vi "LabVIEW_ArduinoControls_TimeProtoType.vi"() -> ()   [LabVIEW 2021]
uses:
  <vilib>/Instr/_visa.llb/VISA Configure Serial Port (Instr).vi
panel:
  out "Horz Distance":dbl(graph)
  out "RPM":dbl(graph)
  out "Vertical Motor Speed":dbl(graph)
  out "Vertical Distance":dbl(graph)
  out "Weight on Bit":dbl(graph)
  out "System Amps":dbl(graph)
  out "RPM":cluster{"X":dbl, "Y":dbl}[](graph)
  out "System Amps":cluster{"X":dbl, "Y":dbl}[](graph)
  out "Horz Distance":cluster{"X":dbl, "Y":dbl}[](graph)
  out "Vertical Distance":cluster{"X":dbl, "Y":dbl}[](graph)
  out "Vertical Motor Speed":cluster{"X":dbl, "Y":dbl}[](graph)
  out "Weight on Bit":cluster{"X":dbl, "Y":dbl}[](graph)
  in  "DRILL STOP":bool
  in  "Drill Speed Arduino 2.0 Write Stop":bool
  in  "Slow Down":bool
  in  "Speed Up":bool
  in  "Drill Speed Arduino 2 Write":refnum<visa-resource-name>
  in  "Stepper Arduino 1 Serial Read":refnum<visa-resource-name>
  out "Data Packet Arduini 1 Matched":i32
  in  "Arduino 1.0 Read Stop":bool
  in  "Arduino 2.0 Read Stop":bool
  in  "Emergency Stop! 3":bool
  in  "Emergency Stop! 2":bool
  in  "GO DOWN 3":bool
  in  "GO DOWN 2":bool
  in  "GO UP 3":bool
  in  "GO UP 2":bool
  in  "MAX SPEED 3":bool
  in  "MAX SPEED 2":bool
  in  "SLOWEST SPEED 3":bool
  in  "SLOWEST SPEED 2":bool
  in  "Decellerate 3":bool
  in  "Decellerate 2":bool
  in  "Accelerate 3":bool
  in  "Accelerate 2":bool
  in  "Drill Speed Arduino 2 Serial Read":refnum<visa-resource-name>
  out "Data Packet Received":i32
  in  "GO UP":bool
  in  "GO DOWN":bool
  in  "MAX SPEED":bool
  in  "SLOWEST SPEED":bool
  out "concatenated string":string
  in  "Arduino 1.0 Write Stop":bool
  in  "Emergency Stop!":bool
  in  "Decellerate":bool
  in  "Stepper Arduino 1 Write":refnum<visa-resource-name>
  in  "Accelerate":bool
  # "Drill Speed Controls"
  # "WINCH CONTROLS"
  # "VERTICAL STEPPER MOTOR CONTROLS"
  # "HORIZONTAL STEPPER MOTOR CONTROLS"
  # "-1 Means Not Found\nany value greater than 0 corresponds to the amount\nof matching characters found"
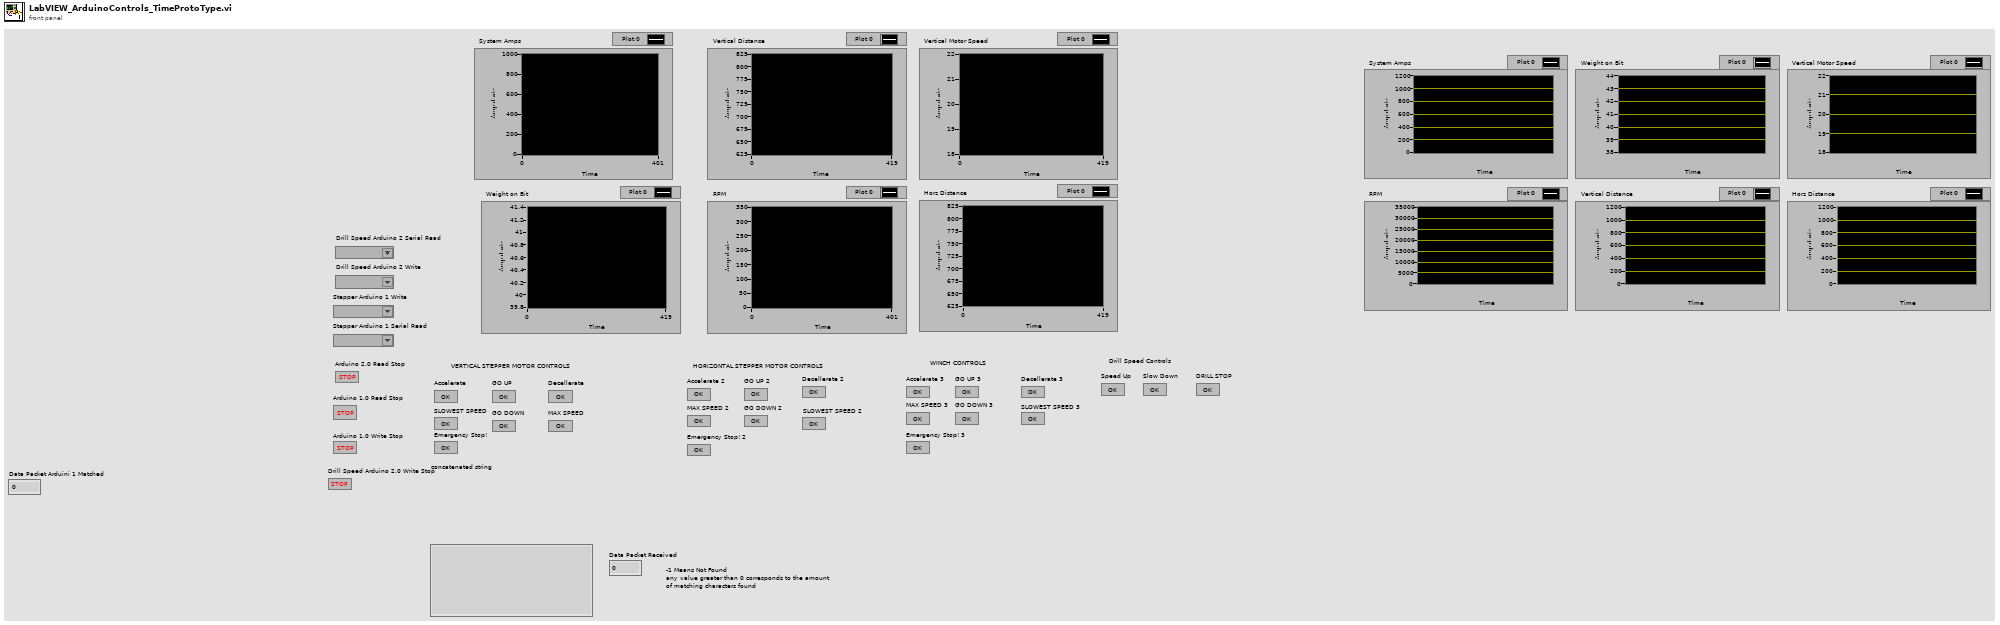
[diagram p1: front panel]
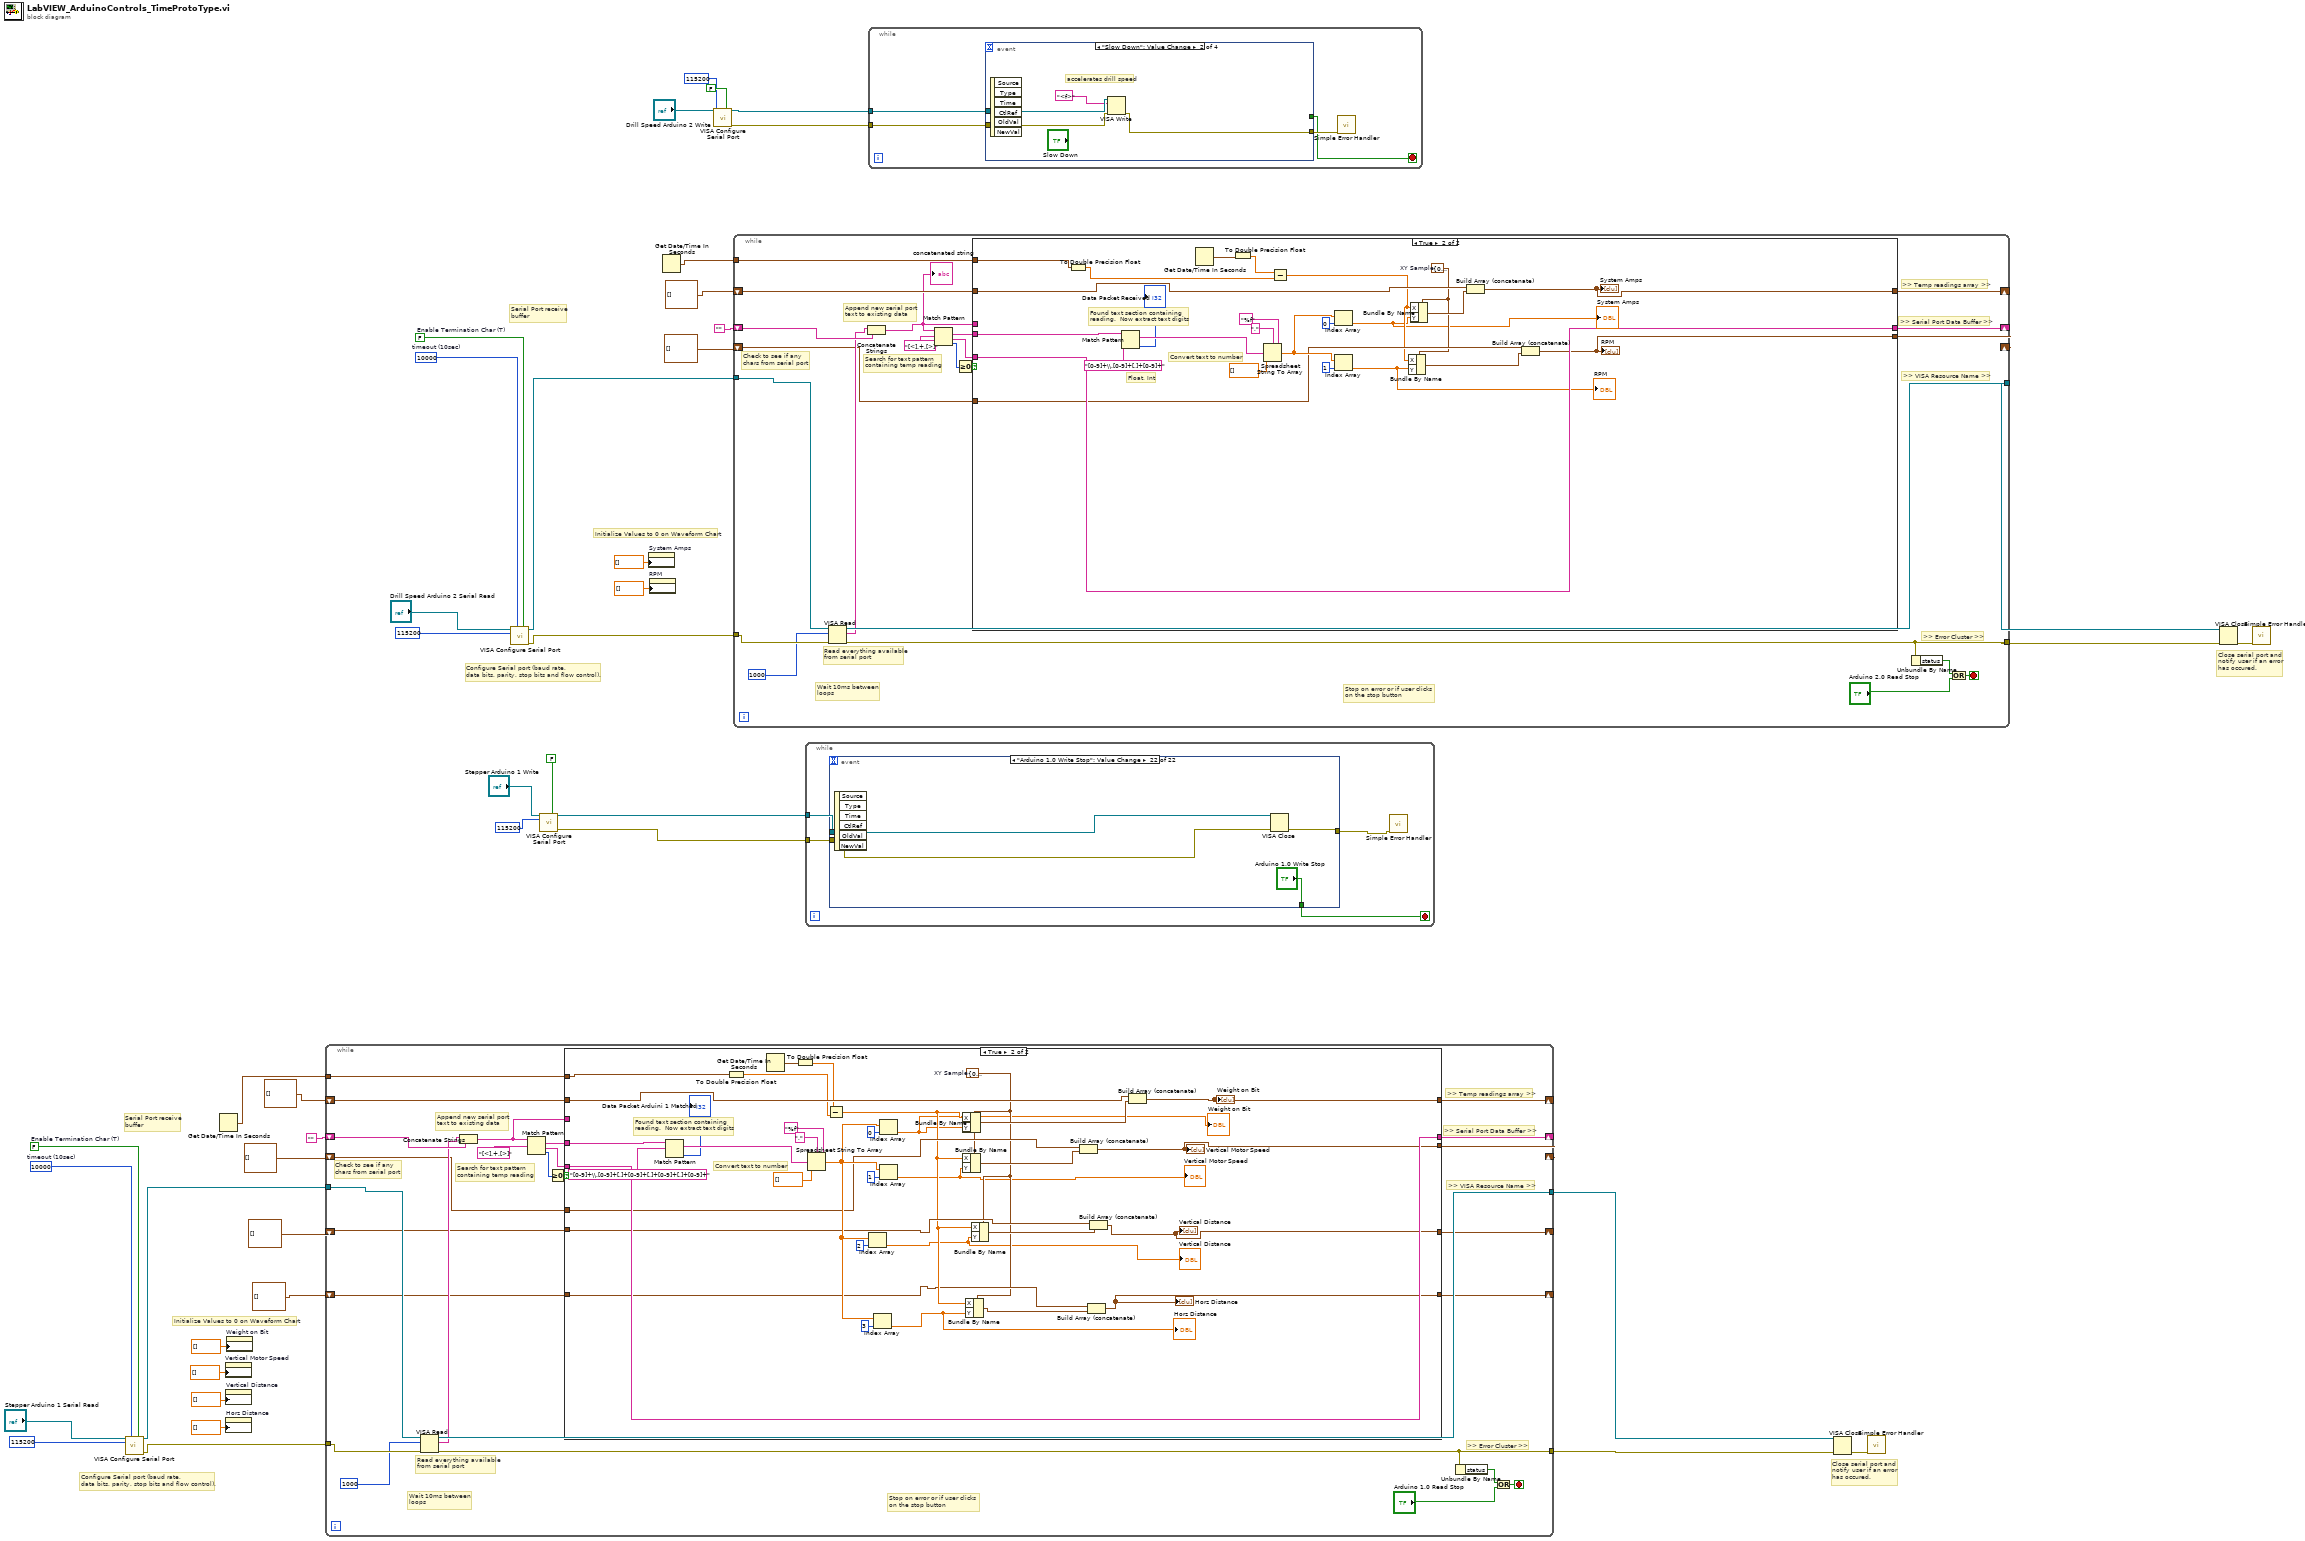
[diagram p0: block diagram]
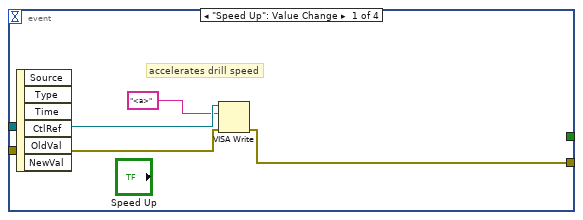
[diagram p2: hidden frame]
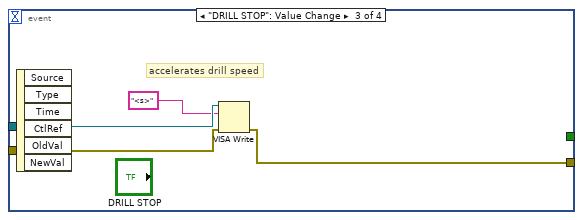
[diagram p3: hidden frame]
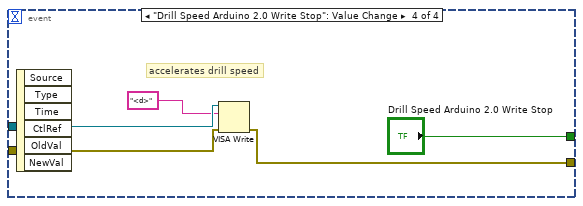
[diagram p4: hidden frame]
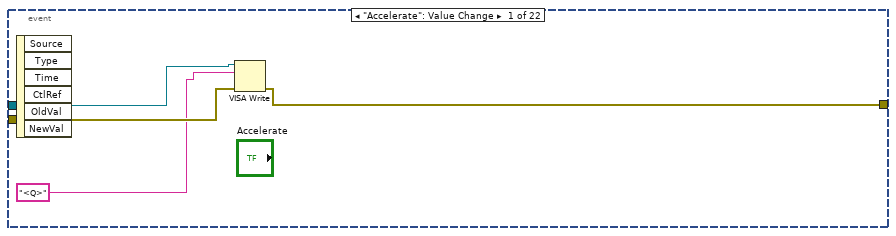
[diagram p7: hidden frame]
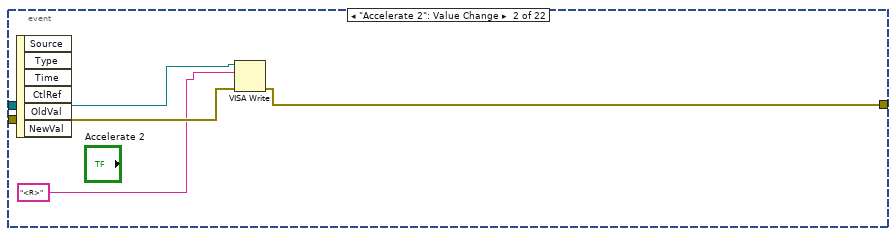
[diagram p8: hidden frame]
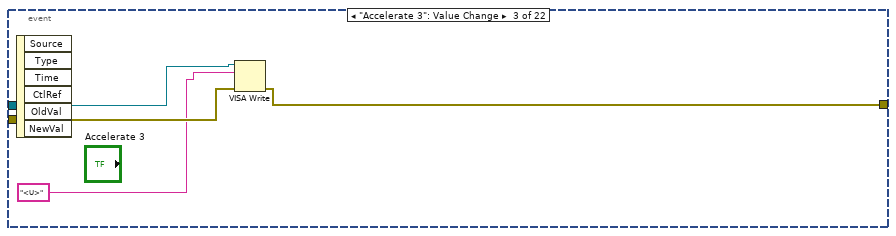
[diagram p9: hidden frame]
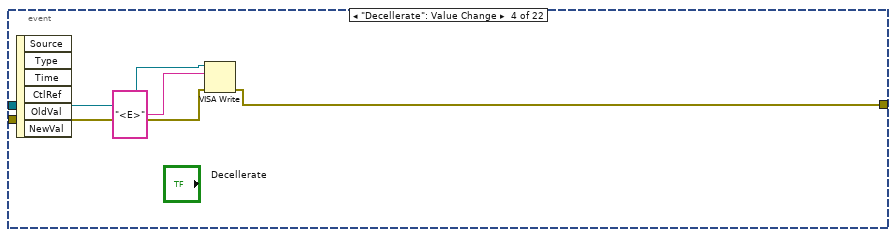
[diagram p10: hidden frame]
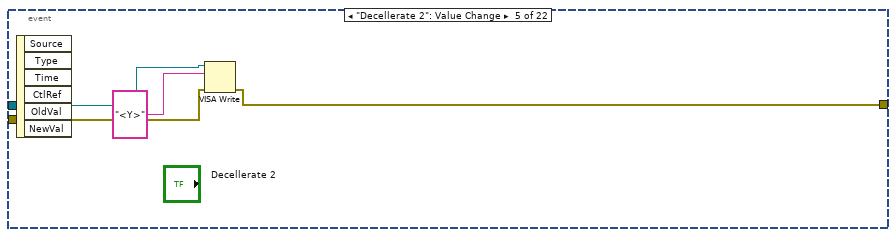
[diagram p11: hidden frame]
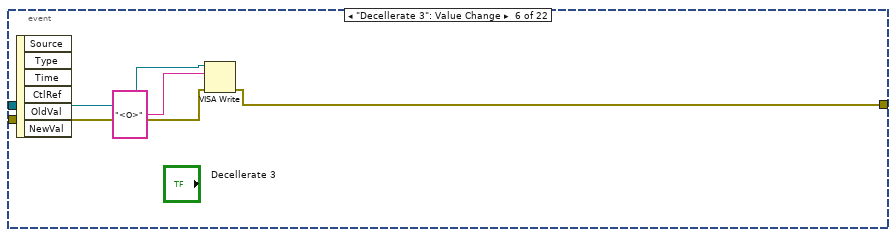
[diagram p12: hidden frame]
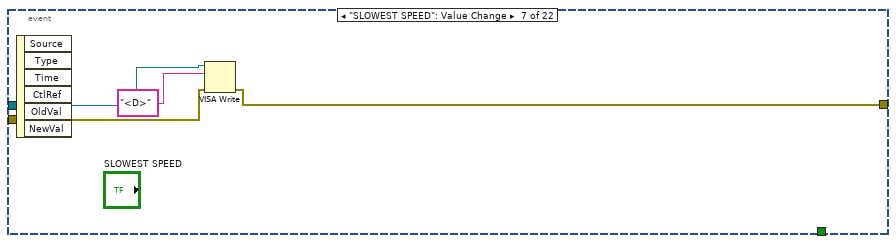
[diagram p13: hidden frame]
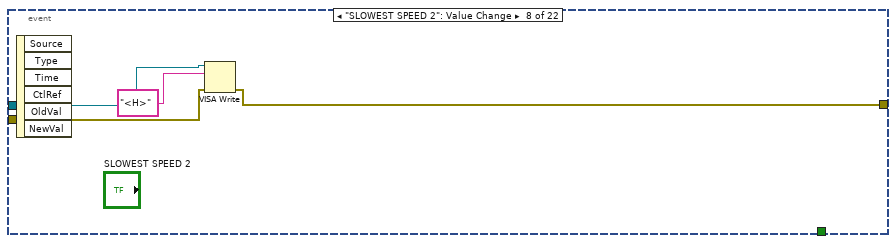
[diagram p14: hidden frame]
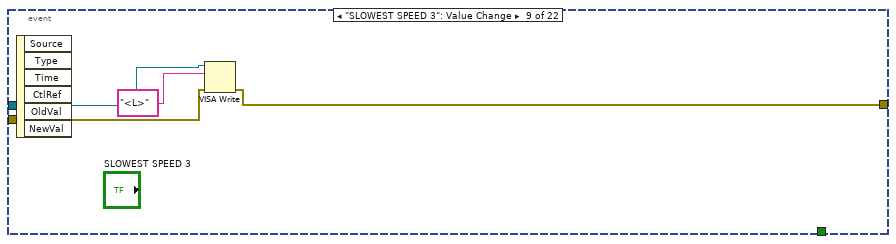
[diagram p15: hidden frame]
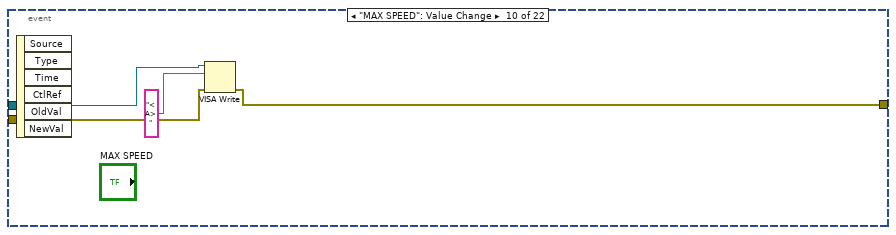
[diagram p16: hidden frame]
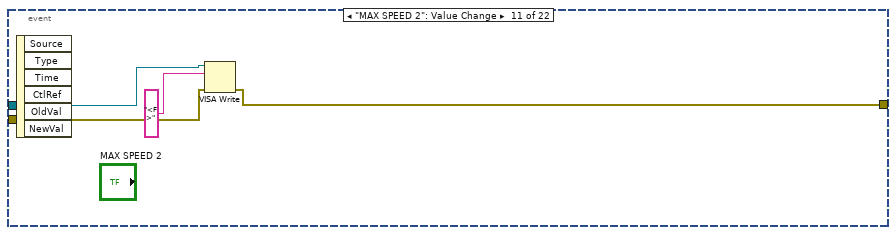
[diagram p17: hidden frame]
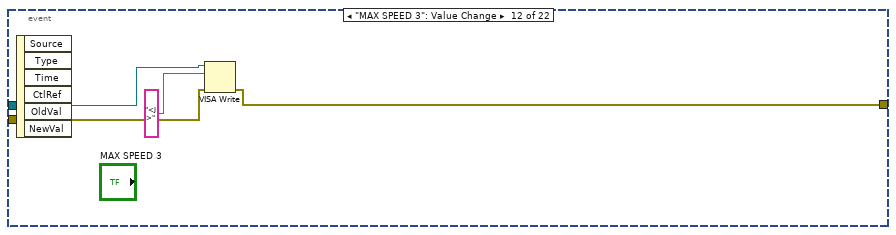
[diagram p18: hidden frame]
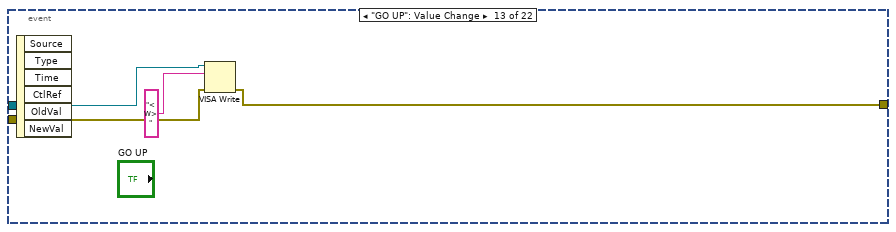
[diagram p19: hidden frame]
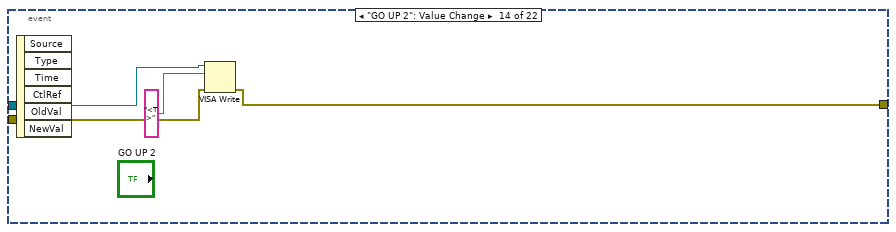
[diagram p20: hidden frame]
diagram:
  w25 = FALSE  # Enable Termination Char (T)
  w26 = u32 10000  # timeout (10sec)
  w36 = FALSE  # Enable Termination Char (T)
  w37 = u32 10000  # timeout (10sec)
  # "Initialize Values to 0 on Waveform Chart"
  # "Initialize Values to 0 on Waveform Chart"
  # "Close serial port and\nnotify user if an error\nhas occured."
  # "Serial Port receive\nbuffer"
  # "Configure Serial port (baud rate,\ndata bits, parity, stop bits and flow control)."
  # "Close serial port and\nnotify user if an error\nhas occured."
  # "Serial Port receive\nbuffer"
  # "Configure Serial port (baud rate,\ndata bits, parity, stop bits and flow control)."
  n1 = call-poly "VISA Configure Serial Port"("VISA resource name"="Stepper Arduino 1 Serial Read", "timeout (10sec)"=w26, "Enable Termination\nChar (T)"=w25, "baud rate (9600)"=u32 115200) -> ("VISA resource name out"=w22:refnum<visa-resource-name>, "error out"=w21:errorcluster)  [unwired: 10 in]
  n2 = Get Date/Time In Seconds() -> (seconds since 1Jan1904=w13:timestamp)
  n3 = property on="Vertical Motor Speed" class="WFChart (strict)"("History Data"=dbl[] []) -> ()  [unwired: 2 in, 2 out]
  n4 = property on="Vertical Distance" class="WFChart (strict)"("History Data"=dbl[] []) -> ()  [unwired: 2 in, 2 out]
  n5 = property on="Horz Distance" class="WFChart (strict)"("History Data"=dbl[] []) -> ()  [unwired: 2 in, 2 out]
  n6 = property on="Weight on Bit" class="WFChart (strict)"("History Data"=dbl[] []) -> ()  [unwired: 2 in, 2 out]
  n7 = while {
    tunnel: [w68] -> w29
    tunnel: [w70] -> w28
    shift-right: [w63] -> _
    shift-left: "" -> [w69]
    shift-right: [w65] -> _
    shift-left: cluster{"X":dbl, "Y":dbl}[] [] ("XY Graph") -> [w64]
    tunnel: w22 -> [w62]
    tunnel: w21 -> [w61]
    shift-right: [w53] -> _
    shift-left: cluster{"X":dbl, "Y":dbl}[] [] ("XY Graph") -> [w52]
    shift-right: [w48] -> _
    shift-left: cluster{"X":dbl, "Y":dbl}[] [] ("XY Graph") -> [w49]
    shift-right: [w46] -> _
    shift-left: cluster{"X":dbl, "Y":dbl}[] [] ("XY Graph") -> [w47]
    tunnel: w13 -> [w45]
    stop <- w67 stop-if-true
    # "Search for text pattern\ncontaining temp reading"
    # "Append new serial port\ntext to existing data"
    # "Read everything available\nfrom serial port"
    # "Wait 10ms between \nloops"
    # "Stop on error or if user clicks \non the stop button"
    # ">> Error Cluster >>"
    # ">> VISA Resource Name >>"
    # ">> Temp readings array >>"
    # ">> Serial Port Data Buffer >>"
    # "Check to see if any\nchars from serial port"
    n8 = VISA Read(VISA resource name=w62, byte count=u32 1000, error in (no error)=w61) -> (VISA resource name out=w70:refnum<visa-resource-name>, read buffer=w55:string, error out=w68:errorcluster)  [unwired: 1 out]
    n9 = Concatenate Strings(w55, w69) -> (w50:string)
    n10 = Match Pattern(string=w50, regular expression="[<].+.[>]") -> (match substring=w57:string, after substring=w56:string, offset past match=w59:i32)  [unwired: 1 in, 1 out]
    n11 = Greater Or Equal To 0?(x=w59) -> (x >= 0?=w58:bool)
    n12 = case shown="True" w58 {
      tunnel: w57 -> [_ w109]
      tunnel: w56 -> [_ w110]
      tunnel: [w73 w110] -> w63
      tunnel: [w75 w96] -> w65
      tunnel: w64 -> [w75 w97]
      tunnel: [w74 w90] -> w53
      tunnel: w52 -> [w74 w89]
      tunnel: w50 -> [w73 _]
      tunnel: w49 -> [w72 w86]
      tunnel: [w72 w87] -> w48
      tunnel: w47 -> [w71 w83]
      tunnel: [w71 w80] -> w46
      tunnel: w45 -> [_ w95]
      frame False {
        # "Did not find text pattern in the buffer.  Try again in the next loop after new data \nhas been received."
      }
      frame True {
        w81 = cluster{"X":dbl, "Y":dbl} {"X"=0.0, "Y"=0.0}  # XY Sample
        # "Convert text to number"
        # "Found text section containing \nreading.  Now extract text digits"
        n13 = Match Pattern(string=w109, regular expression="[0-9]+\\.[0-9]+[,]+[0-9]+[,]+[0-9]+[,]+[0-9]+") -> (match substring=w103:string, offset past match=→"Data Packet Arduini 1 Matched":i32)  [unwired: 1 in, 2 out]
        n14 = To Double Precision Float(number=w95) -> (double precision float=w94:dbl)
        n15 = Get Date/Time In Seconds() -> (seconds since 1Jan1904=w93:timestamp)
        n16 = To Double Precision Float(number=w93) -> (double precision float=w92:dbl)
        n17 = Spreadsheet String To Array(delimiter (Tab)=",", format string="%f", spreadsheet string=w103, array type (2D Dbl)=dbl[] []) -> (array=w99:dbl[])
        n18 = Subtract(x=w92, y=w94) -> (x-y=w84:dbl)
        n19 = Index Array(array=w99, index=2) -> (element=w77:dbl)
        "Vertical Distance" <- w77
        n20 = Index Array(array=w99, index=3) -> (element=w76:dbl)
        "Horz Distance" <- w76
        n21 = Index Array(array=w99, index=0 ("index (row)")) -> (element=w79:dbl)
        "Weight on Bit" <- w79
        n22 = Index Array(array=w99, index=1 ("index (row)")) -> (element=w78:dbl)
        "Vertical Motor Speed" <- w78
        n23 = Bundle By Name(cluster=w81, "X"=w84, "Y"=w79) -> (w91:cluster{"X":dbl, "Y":dbl})
        n24 = Bundle By Name(cluster=w81, "X"=w84, "Y"=w78) -> (w88:cluster{"X":dbl, "Y":dbl})
        n25 = Bundle By Name(cluster=w81, "X"=w84, "Y"=w76) -> (w82:cluster{"X":dbl, "Y":dbl})
        n26 = Bundle By Name(cluster=w81, "X"=w84, "Y"=w77) -> (w85:cluster{"X":dbl, "Y":dbl})
        n27 = Build Array (concatenate)(w89, w88) -> (w90:cluster{"X":dbl, "Y":dbl}[])
        "Vertical Motor Speed" <- w90
        n28 = Build Array (concatenate)(w83, w82) -> (w80:cluster{"X":dbl, "Y":dbl}[])
        "Horz Distance" <- w80
        n29 = Build Array (concatenate)(w86, w85) -> (w87:cluster{"X":dbl, "Y":dbl}[])
        "Vertical Distance" <- w87
        n30 = Build Array (concatenate)(w97, w91) -> (w96:cluster{"X":dbl, "Y":dbl}[])
        "Weight on Bit" <- w96
      }
    }
    n31 = Unbundle By Name(w68) -> ("status"=w66:bool)
    n32 = Or(x=w66, y="Arduino 1.0 Read Stop") -> (x .or. y?=w67:bool)
  }
  n33 = call-poly "VISA Configure Serial Port"("VISA resource name"="Drill Speed Arduino 2 Serial Read", "timeout (10sec)"=w37, "Enable Termination\nChar (T)"=w36, "baud rate (9600)"=u32 115200) -> ("VISA resource name out"=w33:refnum<visa-resource-name>, "error out"=w32:errorcluster)  [unwired: 10 in]
  n34 = call-poly "VISA Configure Serial Port"("VISA resource name"="Stepper Arduino 1 Write", "Enable Termination\nChar (T)"=FALSE ("Enable Termination\nChar (T)"), "baud rate (9600)"=u32 115200) -> ("VISA resource name out"=w44:refnum<visa-resource-name>, "error out"=w43:errorcluster)  [unwired: 11 in]
  n35 = property on="System Amps" class="WFChart (strict)"("History Data"=dbl[] []) -> ()  [unwired: 2 in, 2 out]
  n36 = property on="RPM" class="WFChart (strict)"("History Data"=dbl[] []) -> ()  [unwired: 2 in, 2 out]
  n37 = Get Date/Time In Seconds() -> (seconds since 1Jan1904=w9:timestamp)
  n38 = call-poly "VISA Configure Serial Port"("VISA resource name"="Drill Speed Arduino 2 Write", "Enable Termination\nChar (T)"=FALSE ("Enable Termination\nChar (T)"), "baud rate (9600)"=u32 115200) -> ("VISA resource name out"=w19:refnum<visa-resource-name>, "error out"=w18:errorcluster)  [unwired: 11 in]
  n39 = while {
    tunnel: [w130] -> w40
    tunnel: [w132] -> w39
    shift-right: [w125] -> _
    shift-left: "" -> [w131]
    shift-right: [w127] -> _
    shift-left: cluster{"X":dbl, "Y":dbl}[] [] ("XY Graph") -> [w126]
    tunnel: w33 -> [w124]
    tunnel: w32 -> [w123]
    shift-right: [w115] -> _
    shift-left: cluster{"X":dbl, "Y":dbl}[] [] ("XY Graph") -> [w114]
    tunnel: w9 -> [w111]
    stop <- w129 stop-if-true
    # "Search for text pattern\ncontaining temp reading"
    # "Append new serial port\ntext to existing data"
    # "Read everything available\nfrom serial port"
    # "Wait 10ms between \nloops"
    # "Stop on error or if user clicks \non the stop button"
    # ">> Error Cluster >>"
    # ">> VISA Resource Name >>"
    # ">> Temp readings array >>"
    # ">> Serial Port Data Buffer >>"
    # "Check to see if any\nchars from serial port"
    n40 = VISA Read(VISA resource name=w124, byte count=u32 1000, error in (no error)=w123) -> (VISA resource name out=w132:refnum<visa-resource-name>, read buffer=w117:string, error out=w130:errorcluster)  [unwired: 1 out]
    n41 = Concatenate Strings(w117, w131) -> (w112:string)
    "concatenated string" <- w112
    n42 = Match Pattern(string=w112, regular expression="[<].+.[>]") -> (match substring=w119:string, after substring=w118:string, offset past match=w121:i32)  [unwired: 1 in, 1 out]
    n43 = Greater Or Equal To 0?(x=w121) -> (x >= 0?=w120:bool)
    n44 = case shown="True" w120 {
      tunnel: w119 -> [_ w159]
      tunnel: w118 -> [_ w160]
      tunnel: [w133 w160] -> w125
      tunnel: [w135 w149] -> w127
      tunnel: w126 -> [w135 w144]
      tunnel: [w134 w142] -> w115
      tunnel: w114 -> [w134 w141]
      tunnel: w112 -> [w133 _]
      tunnel: w111 -> [_ w148]
      frame False {
        # "Did not find text pattern in the buffer.  Try again in the next loop after new data \nhas been received."
      }
      frame True {
        w138 = cluster{"X":dbl, "Y":dbl} {"X"=0.0, "Y"=0.0}  # XY Sample
        # "Float, Int"
        # "Convert text to number"
        # "Found text section containing \nreading.  Now extract text digits"
        n45 = To Double Precision Float(number=w148) -> (double precision float=w146:dbl)
        n46 = Match Pattern(string=w159, regular expression="[0-9]+\\.[0-9]+[,]+[0-9]+") -> (match substring=w153:string, offset past match=→"Data Packet Received":i32)  [unwired: 1 in, 2 out]
        n47 = Get Date/Time In Seconds() -> (seconds since 1Jan1904=w147:timestamp)
        n48 = To Double Precision Float(number=w147) -> (double precision float=w145:dbl)
        n49 = Spreadsheet String To Array(delimiter (Tab)=",", format string="%f", spreadsheet string=w153, array type (2D Dbl)=dbl[] []) -> (array=w150:dbl[])
        n50 = Subtract(x=w145, y=w146) -> (x-y=w140:dbl)
        n51 = Index Array(array=w150, index=0 ("index (row)")) -> (element=w136:dbl)
        "System Amps" <- w136
        n52 = Index Array(array=w150, index=1 ("index (row)")) -> (element=w137:dbl)
        "RPM" <- w137
        n53 = Bundle By Name(cluster=w138, "X"=w140, "Y"=w137) -> (w139:cluster{"X":dbl, "Y":dbl})
        n54 = Bundle By Name(cluster=w138, "X"=w140, "Y"=w136) -> (w143:cluster{"X":dbl, "Y":dbl})
        n55 = Build Array (concatenate)(w144, w143) -> (w149:cluster{"X":dbl, "Y":dbl}[])
        "System Amps" <- w149
        n56 = Build Array (concatenate)(w141, w139) -> (w142:cluster{"X":dbl, "Y":dbl}[])
        "RPM" <- w142
      }
    }
    n57 = Unbundle By Name(w130) -> ("status"=w128:bool)
    n58 = Or(x=w128, y="Arduino 2.0 Read Stop") -> (x .or. y?=w129:bool)
  }
  n59 = while {
    tunnel: w44 -> [w164]
    tunnel: w43 -> [w163]
    stop <- w161 stop-if-true
    n60 = event shown="[21] \"Arduino 1.0 Write Stop\": Value Change" {
      selector: _ -> [_ _ _ _ _ _ _ _ _ _ _ _ _ _ _ _ _ _ _ _ _ _]
      dyn-events: _ -> [_ _ _ _ _ _ _ _ _ _ _ _ _ _ _ _ _ _ _ _ _ _]
      timeout: _ -> [_ _ _ _ _ _ _ _ _ _ _ _ _ _ _ _ _ _ _ _ _ _]
      tunnel: [w168 w172 w176 w180 w184 w188 w192 w196 w200 w204 w208 w212 w216 w220 w224 w228 w232 w236 w240 w244 w248 w252] -> w162
      tunnel: w164 -> [w167 w171 w175 w178 w182 w186 w190 w194 w198 w202 w206 w210 w214 w218 w222 w226 w230 w234 w238 w242 w246 w251]
      tunnel: w163 -> [w166 w170 w174 w177 w181 w185 w189 w193 w197 w201 w205 w209 w213 w217 w221 w225 w229 w233 w237 w241 w245 w250]
      tunnel: [_ _ _ _ _ _ _ _ _ _ _ _ _ _ _ _ _ _ _ _ _ "Arduino 1.0 Write Stop"] -> w161
      event "Accelerate": Value Change {
        n61 = event-data() -> ()  [unwired: 1 in, 6 out]
        n62 = VISA Write(VISA resource name=w167, write buffer="<Q>", error in (no error)=w166) -> (error out=w168:errorcluster)  [unwired: 2 out]
      }
      event "Accelerate 2": Value Change {
        n63 = event-data() -> ()  [unwired: 1 in, 6 out]
        n64 = VISA Write(VISA resource name=w171, write buffer="<R>", error in (no error)=w170) -> (error out=w172:errorcluster)  [unwired: 2 out]
      }
      event "Accelerate 3": Value Change {
        n65 = event-data() -> ()  [unwired: 1 in, 6 out]
        n66 = VISA Write(VISA resource name=w175, write buffer="<U>", error in (no error)=w174) -> (error out=w176:errorcluster)  [unwired: 2 out]
      }
      event "Decellerate": Value Change {
        n67 = event-data() -> ()  [unwired: 1 in, 6 out]
        n68 = VISA Write(VISA resource name=w178, write buffer="<E>", error in (no error)=w177) -> (error out=w180:errorcluster)  [unwired: 2 out]
      }
      event "Decellerate 2": Value Change {
        n69 = event-data() -> ()  [unwired: 1 in, 6 out]
        n70 = VISA Write(VISA resource name=w182, write buffer="<Y>", error in (no error)=w181) -> (error out=w184:errorcluster)  [unwired: 2 out]
      }
      event "Decellerate 3": Value Change {
        n71 = event-data() -> ()  [unwired: 1 in, 6 out]
        n72 = VISA Write(VISA resource name=w186, write buffer="<O>", error in (no error)=w185) -> (error out=w188:errorcluster)  [unwired: 2 out]
      }
      event "SLOWEST SPEED": Value Change {
        n73 = event-data() -> ()  [unwired: 1 in, 6 out]
        n74 = VISA Write(VISA resource name=w190, write buffer="<D>", error in (no error)=w189) -> (error out=w192:errorcluster)  [unwired: 2 out]
      }
      event "SLOWEST SPEED 2": Value Change {
        n75 = event-data() -> ()  [unwired: 1 in, 6 out]
        n76 = VISA Write(VISA resource name=w194, write buffer="<H>", error in (no error)=w193) -> (error out=w196:errorcluster)  [unwired: 2 out]
      }
      event "SLOWEST SPEED 3": Value Change {
        n77 = event-data() -> ()  [unwired: 1 in, 6 out]
        n78 = VISA Write(VISA resource name=w198, write buffer="<L>", error in (no error)=w197) -> (error out=w200:errorcluster)  [unwired: 2 out]
      }
      event "MAX SPEED": Value Change {
        n79 = event-data() -> ()  [unwired: 1 in, 6 out]
        n80 = VISA Write(VISA resource name=w202, write buffer="<A>", error in (no error)=w201) -> (error out=w204:errorcluster)  [unwired: 2 out]
      }
      event "MAX SPEED 2": Value Change {
        n81 = event-data() -> ()  [unwired: 1 in, 6 out]
        n82 = VISA Write(VISA resource name=w206, write buffer="<F>", error in (no error)=w205) -> (error out=w208:errorcluster)  [unwired: 2 out]
      }
      event "MAX SPEED 3": Value Change {
        n83 = event-data() -> ()  [unwired: 1 in, 6 out]
        n84 = VISA Write(VISA resource name=w210, write buffer="<J>", error in (no error)=w209) -> (error out=w212:errorcluster)  [unwired: 2 out]
      }
      event "GO UP": Value Change {
        n85 = event-data() -> ()  [unwired: 1 in, 6 out]
        n86 = VISA Write(VISA resource name=w214, write buffer="<W>", error in (no error)=w213) -> (error out=w216:errorcluster)  [unwired: 2 out]
      }
      event "GO UP 2": Value Change {
        n87 = event-data() -> ()  [unwired: 1 in, 6 out]
        n88 = VISA Write(VISA resource name=w218, write buffer="<T>", error in (no error)=w217) -> (error out=w220:errorcluster)  [unwired: 2 out]
      }
      event "GO UP 3": Value Change {
        n89 = event-data() -> ()  [unwired: 1 in, 6 out]
        n90 = VISA Write(VISA resource name=w222, write buffer="<I>", error in (no error)=w221) -> (error out=w224:errorcluster)  [unwired: 2 out]
      }
      event "GO DOWN": Value Change {
        n91 = event-data() -> ()  [unwired: 1 in, 6 out]
        n92 = VISA Write(VISA resource name=w226, write buffer="<S>", error in (no error)=w225) -> (error out=w228:errorcluster)  [unwired: 2 out]
      }
      event "GO DOWN 2": Value Change {
        n93 = event-data() -> ()  [unwired: 1 in, 6 out]
        n94 = VISA Write(VISA resource name=w230, write buffer="<G>", error in (no error)=w229) -> (error out=w232:errorcluster)  [unwired: 2 out]
      }
      event "GO DOWN 3": Value Change {
        n95 = event-data() -> ()  [unwired: 1 in, 6 out]
        n96 = VISA Write(VISA resource name=w234, write buffer="<K>", error in (no error)=w233) -> (error out=w236:errorcluster)  [unwired: 2 out]
      }
      event "Emergency Stop!": Value Change {
        n97 = event-data() -> ()  [unwired: 1 in, 6 out]
        n98 = VISA Write(VISA resource name=w238, write buffer="<Z>", error in (no error)=w237) -> (error out=w240:errorcluster)  [unwired: 2 out]
      }
      event "Emergency Stop! 2": Value Change {
        n99 = event-data() -> ()  [unwired: 1 in, 6 out]
        n100 = VISA Write(VISA resource name=w242, write buffer="<C>", error in (no error)=w241) -> (error out=w244:errorcluster)  [unwired: 2 out]
      }
      event "Emergency Stop! 3": Value Change {
        n101 = event-data() -> ()  [unwired: 1 in, 6 out]
        n102 = VISA Write(VISA resource name=w246, write buffer="<N>", error in (no error)=w245) -> (error out=w248:errorcluster)  [unwired: 2 out]
      }
      event "Arduino 1.0 Write Stop": Value Change {
        n103 = event-data() -> ()  [unwired: 1 in, 6 out]
        n104 = VISA Close(VISA resource name=w251, error in (no error)=w250) -> (error out=w252:errorcluster)
      }
    }
    n105 = call <vilib>:"Simple Error Handler.vi"("error in (no error)"=w162) -> ()  [unwired: 4 in, 5 out]
  }
  n106 = while {
    tunnel: w19 -> [w256]
    tunnel: w18 -> [w255]
    stop <- w253 stop-if-true
    n107 = event shown="[1] \"Slow Down\": Value Change" {
      selector: _ -> [_ _ _ _]
      dyn-events: _ -> [_ _ _ _]
      timeout: _ -> [_ _ _ _]
      tunnel: w256 -> [w260 w264 w268 w273]
      tunnel: w255 -> [w259 w263 w267 w272]
      tunnel: [w257 w261 w265 w270] -> w254
      tunnel: [_ _ _ "Drill Speed Arduino 2.0 Write Stop"] -> w253
      event "Speed Up": Value Change {
        # "accelerates drill speed"
        n108 = event-data() -> ()  [unwired: 1 in, 6 out]
        n109 = VISA Write(VISA resource name=w260, write buffer="<a>", error in (no error)=w259) -> (error out=w257:errorcluster)  [unwired: 2 out]
      }
      event "Slow Down": Value Change {
        # "accelerates drill speed"
        n110 = event-data() -> ()  [unwired: 1 in, 6 out]
        n111 = VISA Write(VISA resource name=w264, write buffer="<f>", error in (no error)=w263) -> (error out=w261:errorcluster)  [unwired: 2 out]
      }
      event "DRILL STOP": Value Change {
        # "accelerates drill speed"
        n112 = event-data() -> ()  [unwired: 1 in, 6 out]
        n113 = VISA Write(VISA resource name=w268, write buffer="<s>", error in (no error)=w267) -> (error out=w265:errorcluster)  [unwired: 2 out]
      }
      event "Drill Speed Arduino 2.0 Write Stop": Value Change {
        # "accelerates drill speed"
        n114 = event-data() -> ()  [unwired: 1 in, 6 out]
        n115 = VISA Write(VISA resource name=w273, write buffer="<d>", error in (no error)=w272) -> (error out=w270:errorcluster)  [unwired: 2 out]
      }
    }
    n116 = call <vilib>:"Simple Error Handler.vi"("error in (no error)"=w254) -> ()  [unwired: 4 in, 5 out]
  }
  n117 = VISA Close(VISA resource name=w28, error in (no error)=w29) -> (error out=w27:errorcluster)
  n118 = call <vilib>:"Simple Error Handler.vi"("error in (no error)"=w27) -> ()  [unwired: 4 in, 5 out]
  n119 = VISA Close(VISA resource name=w39, error in (no error)=w40) -> (error out=w38:errorcluster)
  n120 = call <vilib>:"Simple Error Handler.vi"("error in (no error)"=w38) -> ()  [unwired: 4 in, 5 out]
